vi "Build Table.vi"(3 "Row.Headers":string[](array[string]), 4 "Column.Headers":string[](array[string]), 5 "Table.Data.Text":string[][](array[string])) -> (0 "Column.Headers":bool, 1 "Row.Headers":bool, 2 "Table.Text":string[][](array[string]))   [LabVIEW 2017, in "Word_Specific.lvlib" / "xwpfTable.lvclass"]
uses:
  xwpfTable.lvclass
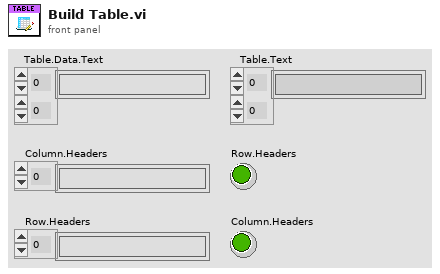
[diagram p1: front panel]
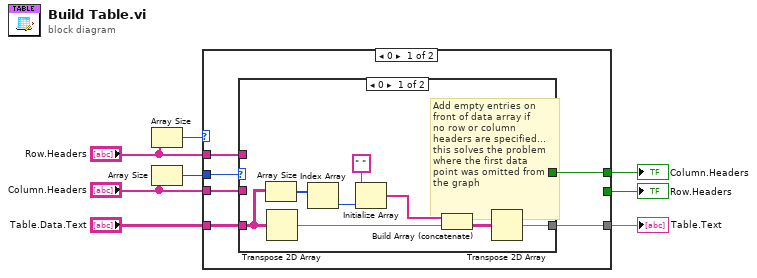
[diagram p0: block diagram]
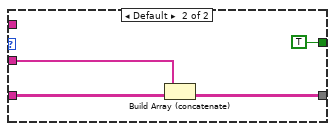
[diagram p2: hidden frame]
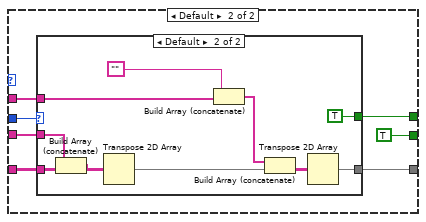
[diagram p3: hidden frame]
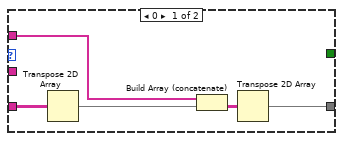
[diagram p4: hidden frame]
diagram:
  n1 = Array Size(array="Row.Headers") -> (size(s)=w3:i32)
  n2 = Array Size(array="Column.Headers") -> (size(s)=w4:i32)
  n3 = case shown="0" w3 {
    tunnel: "Table.Data.Text" -> [w14 w32]
    tunnel: "Column.Headers" -> [w13 w31]
    tunnel: "Row.Headers" -> [w12 w33]
    tunnel: [w11 w29] -> w5
    tunnel: w4 -> [w10 w30]
    tunnel: [_ TRUE] -> w2
    tunnel: [w9 w27] -> w1
    frame 0 {
      n4 = case shown="0" w10 {
        tunnel: w13 -> [_ w26]
        tunnel: w14 -> [w19 w25]
        tunnel: [w20 w24] -> w11
        tunnel: w12 -> [_ _]
        tunnel: [_ TRUE] -> w9
        frame 0 {
          # "Add empty entries on\nfront of data array if\nno row or column \nheaders are specified...\nthis solves the problem\nwhere the first data \npoint was omitted from\nthe graph"
          n5 = Array Size(array=w19) -> (size(s)=w18:i32[])
          n6 = Transpose 2D Array(2D array=w19) -> (transposed array=w21:string[][])
          n7 = Index Array(array=w18) -> (element=w17:i32)  [unwired: 1 in]
          n8 = Initialize Array(" ", w17) -> (w16:string[])
          n9 = Build Array (concatenate)(w16, w21) -> (w22:string[][])
          n10 = Transpose 2D Array(2D array=w22) -> (transposed array=w20:string[][])
        }
        frame Default {
          n11 = Build Array (concatenate)(w26, w25) -> (w24:string[][])
        }
      }
    }
    frame Default {
      n12 = case shown="Default" w30 {
        tunnel: [w35 w46] -> w29
        tunnel: w31 -> [_ w43]
        tunnel: w32 -> [w37 w42]
        tunnel: w33 -> [w38 w40]
        tunnel: [_ TRUE] -> w27
        frame 0 {
          n13 = Transpose 2D Array(2D array=w37) -> (transposed array=w36:string[][])
          n14 = Build Array (concatenate)(w38, w36) -> (w34:string[][])
          n15 = Transpose 2D Array(2D array=w34) -> (transposed array=w35:string[][])
        }
        frame Default {
          n16 = Build Array (concatenate)(w43, w42) -> (w41:string[][])
          n17 = Transpose 2D Array(2D array=w41) -> (transposed array=w45:string[][])
          n18 = Build Array (concatenate)("", w40) -> (w44:string[])
          n19 = Build Array (concatenate)(w44, w45) -> (w47:string[][])
          n20 = Transpose 2D Array(2D array=w47) -> (transposed array=w46:string[][])
        }
      }
    }
  }
  "Table.Text" <- w5
  "Row.Headers" <- w2
  "Column.Headers" <- w1
